vi "2 BoatInfoToCsvStr.vi"() -> (0 "Log String":string)   [LabVIEW 2011]
doc: "Pulls all data off the global as well as the number of missions we currently have, the number of waypoints, and information about the current waypoint and current status of the goodness functions. Then turns it into a formatted string to be logged."
uses:
  2 Typedefs/logger data.ctl
  2 Typedefs/Which Boat.ctl
  2 Typedefs/UTM Location.ctl
  2 Typedefs/heading.ctl
  2 Typedefs/rate of turn.ctl
  2 Typedefs/robot velocity.ctl
  2 Typedefs/pitch and roll.ctl
  2 Typedefs/generalized sensor status.ctl
  2 Typedefs/indicator LED.ctl
  2 Typedefs/apparent wind direction.ctl
  2 Typedefs/apparent wind speed.ctl
  2 Typedefs/absolute wind direction.ctl
  2 Typedefs/absolute wind speed.ctl
  0x2-OCU-Think Comm/0x2 Typedefs/Current Waypoint.ctl
  2 Typedefs/UTM Circle.ctl
  2 Typedefs/rudder angle.ctl
  2 Typedefs/sail setpt.ctl
  0x2-OCU-Think Comm/0x2 Typedefs/manual override.ctl
  2 Typedefs/setpoints to boat.ctl
  2 Classes/Waypoint/Waypoint.lvclass
  2 Globals/2 Global.vi
  2 Classes/MissionQueue/MissionQueue.lvclass
panel:
  out "String Length":i32
  out "Data Log":T1 {"Current Waypoint Coords"."North" format="%#_10f"; "Current Waypoint Coords"."East" format="%#_8f"; "Robot Pitch/Roll"."Roll" format="%05.1f"; "Robot Pitch/Roll"."Pitch" format="%05.1f"; "Robot\nRate of Turn" format="%05.1f"; "Robot\nHeading" format="%05.1f"; "Robot UTM Location"."North" format="%#_10f"; "Robot UTM Location"."East" format="%#_8f"}
  # "Where Am I?"
  # "Path Planning"
  # "From Planning Functions"
  # "(this is not a cluster because subitems\nare generated in parallel code)"
  # "How Am I?"
  # "What's Around Me?"
  # "As Measured"
  # "As Measured"
  # "Loop Rates"
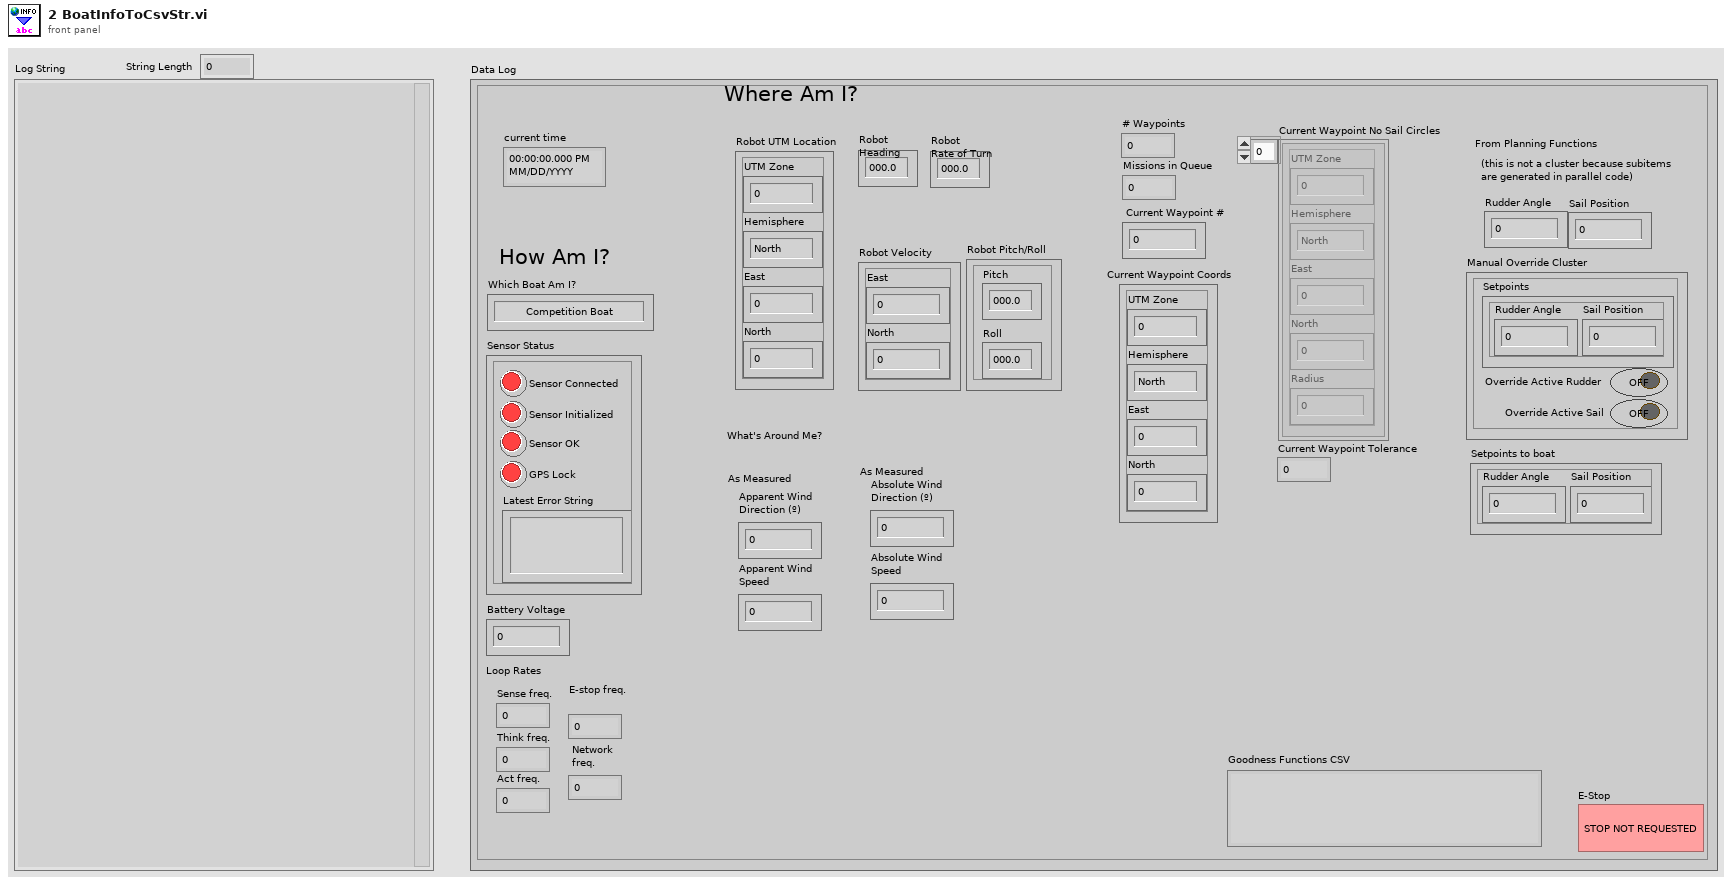
[diagram p1: front panel]
types:
  T1 = typedef "logger data.ctl" = cluster{"current time":timestamp, "Which Boat Am I?":T2, "Robot UTM Location":T3, "Robot\nHeading ":T4, "Robot\nRate of Turn":T5, "Robot Velocity":T6, "Robot Pitch/Roll":T7, "Sensor Status":T8, "Battery Voltage":dbl, "Sense freq.":dbl, "Think freq.":dbl, "Act freq.":dbl, "E-stop freq.":dbl, "Network \nfreq.":dbl, "Apparent Wind\nDirection (º)":T10, "Apparent Wind\nSpeed":T11, "Absolute Wind\nDirection (º)":T12, "Absolute Wind\nSpeed":T13, "Missions in Queue":i32, "# Waypoints":i32, " Current Waypoint #":T14, "Current Waypoint Coords":T3, "Current Waypoint Tolerance":dbl, "Current Waypoint No Sail Circles":T15[], "Rudder Angle":T16, "Sail Position":T17, "Manual Override Cluster":T18, "Setpoints to boat":T19, "E-Stop":bool, "Goodness Functions CSV":string}
  T2 = typedef "Which Boat.ctl" = enum16{"Competition Boat", "Small RC", "Simulation"}
  T3 = typedef "UTM Location.ctl" = cluster{"UTM Zone":dbl, "Hemisphere":enum16{"North", "South"}, "East":dbl, "North":dbl}
  T4 = typedef "heading.ctl" = dbl
  T5 = typedef "rate of turn.ctl" = dbl
  T6 = typedef "robot velocity.ctl" = cluster{"East":dbl, "North":dbl}
  T7 = typedef "pitch and roll.ctl" = cluster{"Pitch":dbl, "Roll":dbl}
  T8 = typedef "generalized sensor status.ctl" = cluster{"Sensor Connected":T9, "Sensor Initialized":T9, "Sensor OK":T9, "Latest Error String":string, "GPS Lock":T9}
  T9 = typedef "indicator LED.ctl" = bool
  T10 = typedef "apparent wind direction.ctl" = dbl
  T11 = typedef "apparent wind speed.ctl" = dbl
  T12 = typedef "absolute wind direction.ctl" = dbl
  T13 = typedef "absolute wind speed.ctl" = dbl
  T14 = typedef "Current Waypoint.ctl" = i32
  T15 = typedef "UTM Circle.ctl" = cluster{"UTM Zone":dbl, "Hemisphere":enum16{"North", "South"}, "East":dbl, "North":dbl, "Radius":dbl}
  T16 = typedef "rudder angle.ctl" = dbl
  T17 = typedef "sail setpt.ctl" = dbl
  T18 = typedef "manual override.ctl" = cluster{"Override Active Rudder":bool, "Setpoints":T19, "Override Active Sail":bool}
  T19 = typedef "setpoints to boat.ctl" = cluster{"Sail Position":T17, "Rudder Angle":T16}
  T20 = typedef "Waypoints List.ctl" = refnum<class "Waypoint.lvclass">[]
  T21 = typedef "Goodness Fns Indicator.ctl" = cluster{dbl, dbl, dbl[][]}
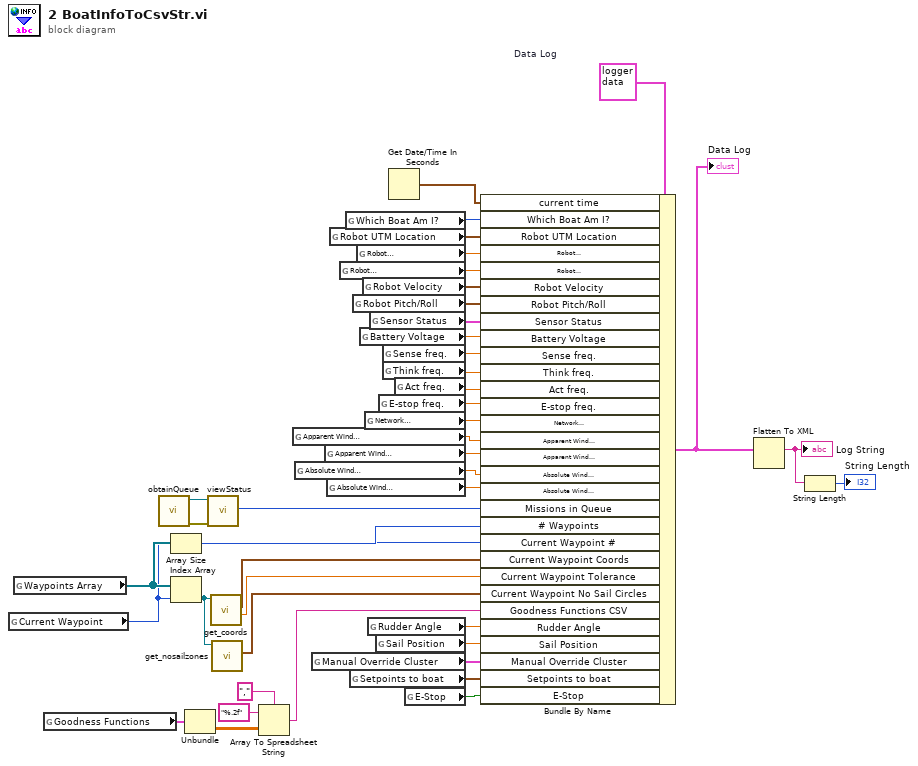
[diagram p0: block diagram]
diagram:
  w38 = T1 {"current time"=timestamp(0 s since 1904-01-01), "Which Boat Am I?"=enum."Competition Boat", "Robot UTM Location"={"UTM Zone"=0.0, "Hemisphere"=enum."North", "East"=0.0, "North"=0.0}, "Robot\nHeading "=0.0, "Robot\nRate of Turn"=0.0, "Robot Velocity"={"East"=0.0, "North"=0.0}, "Robot Pitch/Roll"={"Pitch"=0.0, "Roll"=0.0}, "Sensor Status"={"Sensor Connected"=FALSE, "Sensor Initialized"=FALSE, "Sensor OK"=FALSE, "Latest Error String"="", "GPS Lock"=FALSE}, "Battery Voltage"=0.0, "Sense freq."=0.0, "Think freq."=0.0, "Act freq."=0.0, "E-stop freq."=0.0, "Network \nfreq."=0.0, "Apparent Wind\nDirection (º)"=0.0, "Apparent Wind\nSpeed"=0.0, "Absolute Wind\nDirection (º)"=0.0, "Absolute Wind\nSpeed"=0.0, "Missions in Queue"=0, "# Waypoints"=0, " Current Waypoint #"=0, "Current Waypoint Coords"={"UTM Zone"=0.0, "Hemisphere"=enum."North", "East"=0.0, "North"=0.0}, "Current Waypoint Tolerance"=0.0, "Current Waypoint No Sail Circles"=[], "Rudder Angle"=0.0, "Sail Position"=0.0, "Manual Override Cluster"={"Override Active Rudder"=FALSE, "Setpoints"={"Sail Position"=0.0, "Rudder Angle"=0.0}, "Override Active Sail"=FALSE}, "Setpoints to boat"={"Sail Position"=0.0, "Rudder Angle"=0.0}, "E-Stop"=FALSE, "Goodness Functions CSV"=""}  # Data Log
  n1 = global read "2 Global.vi" "Current Waypoint"() -> (w36:T14)
  n2 = global read "2 Global.vi" "Waypoints Array"() -> (w41:T20)
  n3 = global read "2 Global.vi" "Goodness Functions"() -> (w5:T21)
  n4 = call "obtainQueue.vi"() -> ("Error Out"=w39:errorcluster, "MissionQueue.lvclass"=w40:refnum<class "MissionQueue.lvclass">)  [unwired: 10 in]
  n5 = Array Size(array=w41) -> (size(s)=w37:i32)
  n6 = Index Array(array=w41, index=w36) -> (element=w42:refnum<class "Waypoint.lvclass">)
  n7 = Unbundle(w5) -> (w4:dbl[][])  [unwired: 2 out]
  n8 = call "viewStatus.vi"("error in (no error)"=w39, "MissionQueue in"=w40) -> ("Queue length"=w25:i32)  [unwired: 6 in, 3 out]
  n9 = call-dynamic "get_coords.vi"("Waypoint in"=w42) -> ("Tolerance (meters?)"=w34:dbl, "Coords"=w35:T3)  [unwired: 7 in, 2 out]
  n10 = call-dynamic "get_nosailzones.vi"("Waypoint in"=w42) -> ("No Sail Circles"=w33:T15[])  [unwired: 7 in, 2 out]
  n11 = Array To Spreadsheet String(delimiter (Tab)=",", array=w4, 3:"%.2f" ("format string")) -> (spreadsheet string=w1:string)
  n12 = global read "2 Global.vi" "Apparent Wind\nDirection (º)"() -> (w21:T10)
  n13 = global read "2 Global.vi" "Absolute Wind\nDirection (º)"() -> (w24:T12)
  n14 = global read "2 Global.vi" "Manual Override Cluster"() -> (w28:T18)
  n15 = global read "2 Global.vi" "Apparent Wind\nSpeed"() -> (w22:T11)
  n16 = global read "2 Global.vi" "Absolute Wind\nSpeed"() -> (w23:T13)
  n17 = global read "2 Global.vi" "Robot UTM Location"() -> (w31:T3)
  n18 = global read "2 Global.vi" "Robot\nRate of Turn"() -> (w11:T5)
  n19 = global read "2 Global.vi" "Which Boat Am I?"() -> (w9:T2)
  n20 = global read "2 Global.vi" "Setpoints to boat"() -> (w29:T19)
  n21 = global read "2 Global.vi" "Robot Pitch/Roll"() -> (w13:T7)
  n22 = global read "2 Global.vi" "Robot\nHeading"() -> (w10:T4)
  n23 = global read "2 Global.vi" "Battery Voltage"() -> (w15:dbl)
  n24 = global read "2 Global.vi" "Robot Velocity"() -> (w12:T6)
  n25 = global read "2 Global.vi" "Network \nfreq."() -> (w20:dbl)
  n26 = global read "2 Global.vi" "Rudder Angle"() -> (w26:T16)
  n27 = global read "2 Global.vi" "Sensor Status"() -> (w14:T8)
  n28 = global read "2 Global.vi" "Sail Position"() -> (w27:T17)
  n29 = global read "2 Global.vi" "E-stop freq."() -> (w19:dbl)
  n30 = global read "2 Global.vi" "Sense freq."() -> (w16:dbl)
  n31 = global read "2 Global.vi" "Think freq."() -> (w17:dbl)
  n32 = Get Date/Time In Seconds() -> (seconds since 1Jan1904=w32:timestamp)
  n33 = global read "2 Global.vi" "Act freq."() -> (w18:dbl)
  n34 = global read "2 Global.vi" "E-Stop"() -> (w30:bool)
  n35 = Bundle By Name(cluster=w38, "current time"=w32, "Which Boat Am I?"=w9, "Robot UTM Location"=w31, "Robot\nHeading"=w10, "Robot\nRate of Turn"=w11, "Robot Velocity"=w12, "Robot Pitch/Roll"=w13, "Sensor Status"=w14, "Battery Voltage"=w15, "Sense freq."=w16, "Think freq."=w17, "Act freq."=w18, "E-stop freq."=w19, "Network \nfreq."=w20, "Apparent Wind\nDirection (º)"=w21, "Apparent Wind\nSpeed"=w22, "Absolute Wind\nDirection (º)"=w24, "Absolute Wind\nSpeed"=w23, "Missions in Queue"=w25, "# Waypoints"=w37, "Current Waypoint #"=w36, "Current Waypoint Coords"=w35, "Current Waypoint Tolerance"=w34, "Current Waypoint No Sail Circles"=w33, "Goodness Functions CSV"=w1, "Rudder Angle"=w26, "Sail Position"=w27, "Manual Override Cluster"=w28, "Setpoints to boat"=w29, "E-Stop"=w30) -> (w8:T1)
  "Data Log" <- w8
  n36 = Flatten To XML(anything=w8) -> (xml string=w7:string)
  "Log String" <- w7
  n37 = String Length(string=w7) -> (length=→"String Length":i32)
